vi "VI Tree - string.vi"   [LabVIEW 2009]
uses:
  Trim Whitespace/Trim Whitespace (String).vi
  Convert EOLs/Convert EOLs (String).vi
  To Camel Case/To Camel Case (String).vi
  To Proper Case/To Proper Case (String).vi
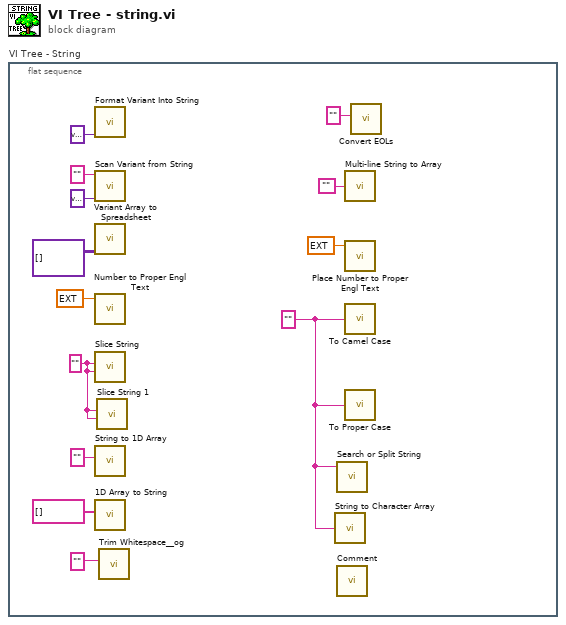
[diagram p0: block diagram]
diagram:
  n1 = flat-sequence "VI Tree - String" {
    frame #0 {
      w1 = "" ("string")
      w2 = "" ("string")
      n2 = call "Format Variant Into String.vi"("Variant"=variant) -> ()  [unwired: 13 in, 2 out]
      n3 = call "Scan Variant from String.vi"("Default Value"=variant, "Input String"="") -> ()  [unwired: 6 in, 4 out]
      n4 = call "Variant Array to Spreadsheet.vi"("2D Variant Array"=variant[][] []) -> ()  [unwired: 9 in, 2 out]
      n5 = call "Number to Proper Engl Text.vi"("Numeric"=ext 0.0) -> ()  [unwired: 4 in, 1 out]
      n6 = call "Slice String.vi"("slice"=w2, "string"=w2) -> ()  [unwired: 5 in, 1 out]
      n7 = call "String to 1D Array.vi"("string"="") -> ()  [unwired: 10 in, 1 out]
      n8 = call "1D Array to String.vi"("Array of Strings"=string[] []) -> ()  [unwired: 10 in, 1 out]
      n9 = call "Slice String 1.vi"("Subset (i:j)"=w2, "String"=w2) -> ()  [unwired: 7 in, 1 out]
      n10 = call-poly "Trim Whitespace__og.vi"("String in"="") -> ()  [unwired: 6 in, 1 out]
      n11 = call "String to Character Array.vi"("Input String"=w1) -> ()  [unwired: 1 out]
      n12 = call "Search or Split String.vi"("string"=w1) -> ()  [unwired: 2 in, 3 out]
      n13 = call "Comment.vi"() -> ()  [unwired: 1 in]
      n14 = call "Multi-line String to Array.vi"("string"="") -> ()  [unwired: 1 out]
      n15 = call "Place Number to Proper Engl Text.vi"("Numeric"=ext 0.0) -> ()  [unwired: 4 in, 1 out]
      n16 = call-poly "To Camel Case.vi"("string"=w1) -> ()  [unwired: 1 in, 1 out]
      n17 = call-poly "To Proper Case.vi"("string"=w1) -> ()  [unwired: 4 in, 1 out]
      n18 = call-poly "Convert EOLs.vi"("String in"="") -> ()  [unwired: 10 in, 1 out]
    }
  }
